vi "NewConcreteCreatorA.vi"(8 "error in (no error)":errorcluster) -> (0 "error out":errorcluster, 3 "ConcreteCreatorA out":refnum<class "ConcreteCreatorA.lvclass">)   [LabVIEW 2020, in "FactoryMethod.lvlib" / "ConcreteCreatorA.lvclass"]
uses:
  ConcreteCreatorA.lvclass
  ConcreteCreatorA.lvclass/ConcreteCreatorA.ctl
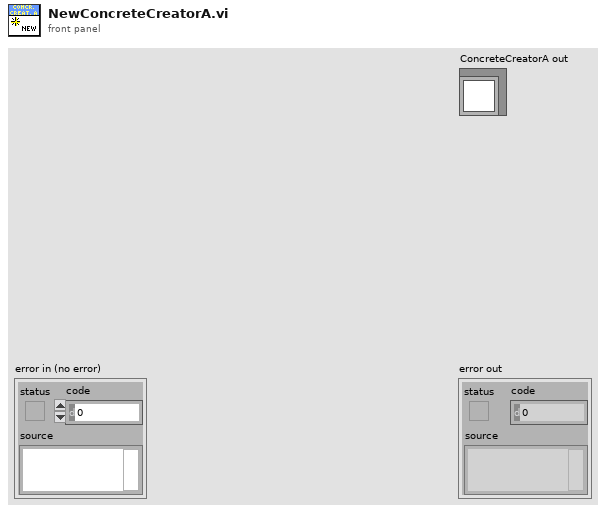
[diagram p1: front panel]
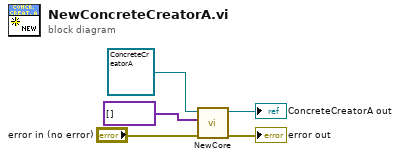
[diagram p0: block diagram]
diagram:
  n1 = call-dynamic "NewCore.vi"("error in (no error)"="error in (no error)", "ParamsArray"=variant[] [], "ConcreteCreatorA in"=refnum<class "ConcreteCreatorA.lvclass"> refnum) -> ("error out"=→"error out":errorcluster, "ConcreteCreatorA out"=→"ConcreteCreatorA out":refnum<class "ConcreteCreatorA.lvclass">)  [unwired: 7 in]
